vi "GetParent_Root_ReturnsError.vi"() -> (0 "error out":errorcluster)   [LabVIEW 2019, in "ResultTreeTest.lvlib"]
uses:
  ResultTreeTest.lvlib
  ResultTree/ResultTree.lvclass
  Assertion/Assertion.lvlib
panel:
  in  "Tree":string(tree)
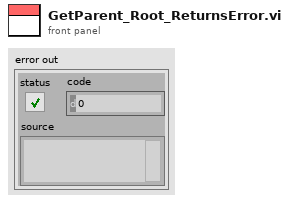
[diagram p1: front panel]
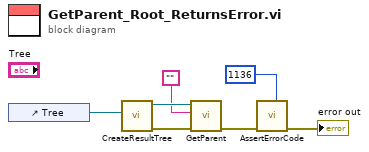
[diagram p0: block diagram]
diagram:
  n1 = control-ref of="Tree"() -> (w6:refnum<vi>)
  n2 = call "CreateResultTree.vi"("Tree Refnum"=w6) -> ("error out"=w5:errorcluster, "ResultTree out"=w4:refnum<class "ResultTree.lvclass">)  [unwired: 9 in]
  n3 = call "GetParent.vi"("error in (no error)"=w5, "Tag"="", "ResultTree in"=w4) -> ("error out"=w3:errorcluster)  [unwired: 6 in, 2 out]
  n4 = call "AssertErrorCode.vi"("Expected"=1136, "error in (no error)"=w3) -> ("error out"=→"error out":errorcluster)  [unwired: 9 in]
